vi "Read commandName.vi"(8 "error in (no error)":errorcluster, 11 "OnInterrupt in":refnum<class "OnInterrupt.lvclass">) -> (0 "error out":errorcluster, 2 "Enum":T1(ring), 3 "OnInterrupt out":refnum<class "OnInterrupt.lvclass">)   [LabVIEW 2016, in "Commands.lvlib" / "OnInterrupt.lvclass"]
uses:
  OnInterrupt.lvclass
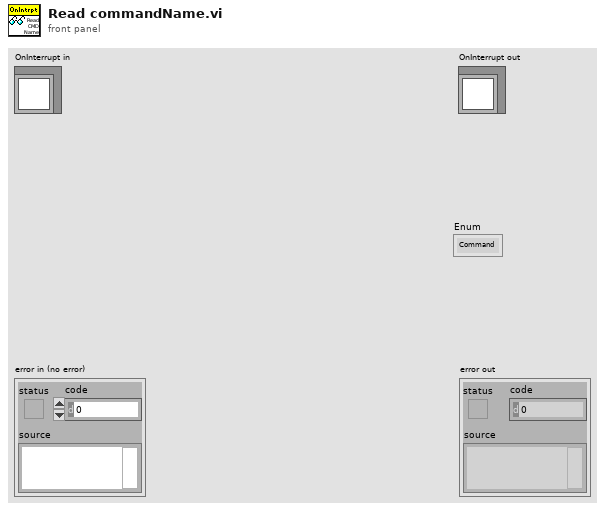
[diagram p1: front panel]
types:
  T1 = enum16{"Command", "Start", "ClearError", "HeartBeat", "Enable", "Disable", "Standby", "Exit", "OnInterrupt", "OnIncomingMessagingError"}
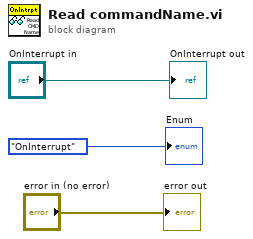
[diagram p0: block diagram]
diagram:
  "error out" <- "error in (no error)"
  "OnInterrupt out" <- "OnInterrupt in"
  "Enum" <- T1."OnInterrupt"
